vi "LabVLC - PauseControl.vi"(3 "error in (no error)":errorcluster, 4 "is_paused":bool, 5 "LabVLC":T1={"media_ptr"=0, "vlc_inst_ptr"=0, "path in"=path "C:/Program Files (x86)/VideoLAN/VLC/libvlc.dll"}) -> (0 "error out":errorcluster, 1 "is_paused":bool, 2 "LabVLC":T1)   [LabVIEW 2014]
doc: "Pause the LabVLC player. If true, the video is paused. If false, the video is playing. Use with a switch for best effect. Requires a LabVLC cluster. The ramifications of calling this function before play are unknown. You may optionally use the boolean output of the pause function to programmatically determine the state of pause."
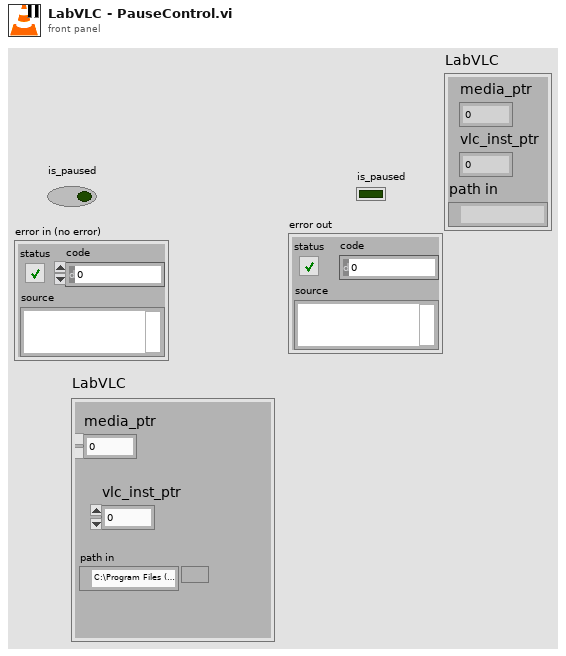
[diagram p1: front panel]
types:
  T1 = cluster{"media_ptr":i32, "vlc_inst_ptr":i32, "path in":path}
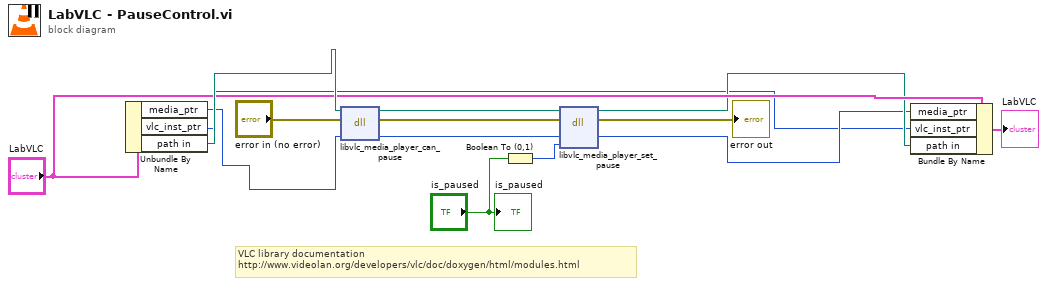
[diagram p0: block diagram]
diagram:
  # "VLC library documentation\nhttp://www.videolan.org/developers/vlc/doc/doxygen/html/modules.html"
  n1 = Unbundle By Name("LabVLC") -> ("media_ptr"=w6:i32, "vlc_inst_ptr"=w2:i32, "path in"=w7:path)
  n2 = dll-call lib="C:/Program Files (x86)/VideoLAN/VLC/libvlc.dll" fn="libvlc_media_player_can_pause"(path in=w7, error in="error in (no error)", "p_mi"=w6) -> (path out=w8:path, error out=w13:errorcluster, "p_mi"=w12:i32)  [unwired: 2 in]
  n3 = Boolean To (0,1)(Boolean="is_paused") -> (0, 1=w11:i16)
  n4 = dll-call lib="C:/Program Files (x86)/VideoLAN/VLC/libvlc.dll" fn="libvlc_media_player_set_pause"(path in=w8, error in=w13, "p_mi"=w12, "do_pause"=w11) -> (path out=w4:path, error out=→"error out":errorcluster, "p_mi"=w3:i32)  [unwired: 3 in]
  n5 = Bundle By Name(cluster="LabVLC", "media_ptr"=w3, "vlc_inst_ptr"=w2, "path in"=w4) -> (→"LabVLC":T1)
  "is_paused" <- "is_paused"
